vi "StartPlay.vi"(8 "error in (no error)":errorcluster, 11 "CameraTestingBL in":refnum<class "CameraTesting.lvclass">) -> (0 "error out":errorcluster, 3 "CameraTestingBL out":refnum<class "CameraTesting.lvclass">)   [LabVIEW 2020, in "CameraTesting.lvlib" / "CameraTesting.lvclass"]
doc: "Send command to camera to starting the data streaming"
uses:
  CameraTesting.lvclass
  CameraTesting.lvclass/CameraTesting.ctl
  <vilib>/ActorFramework/Message Enqueuer/Message Enqueuer.lvclass/Message Enqueuer.ctl
  <vilib>/ActorFramework/Message Enqueuer/Enqueue.vi
  ICameraTestingUI/ICameraTestingUI Messages/StartPlayRslt Msg/StartPlayRslt Msg.lvclass
  C:/Program Files (x86)/National Instruments/LabVIEW 2020/vi.lib/ActorFramework/Message/Message.lvclass
  <vilib>/ActorFramework/Message Priority Queue/Priority Enqueue.vi
  Camera/ICamera/ICamera/ICamera.lvclass
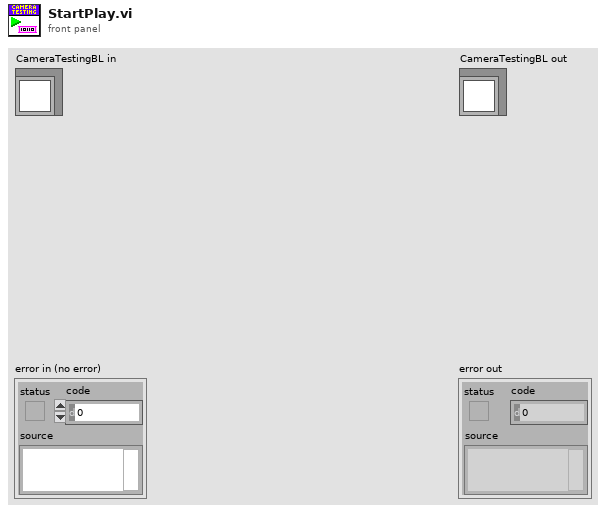
[diagram p1: front panel]
types:
  T1 = typedef "ICameraTesting.lvlib/ICameraTesting.lvclass/StatusUpdated.ctl" = refnum<user-event>
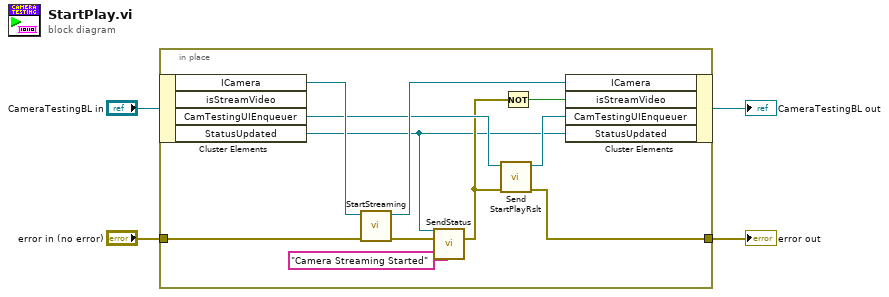
[diagram p0: block diagram]
diagram:
  n1 = in-place {
    in-place-border: "error in (no error)" -> [w15]
    in-place-border: [w10] -> w3
    n2 = in-place-cluster #1("CameraTestingBL in") -> ("ICamera"=w14:refnum<class "ICamera.lvclass">, "CamTestingUIEnqueuer"=w11:refnum<class "Message Enqueuer.lvclass">, "StatusUpdated"=w5:T1)  [unwired: 1 out]
    n3 = call-dynamic "StartStreaming.vi"("error in (no error)"=w15, "ICamera in"=w14) -> ("error out"=w7:errorcluster, "ICamera out"=w13:refnum<class "ICamera.lvclass">)  [unwired: 8 in]
    n4 = call "SendStatus.vi"("StatusUsrEvn"=w5, "error in"=w7, "Text"="Camera Streaming Started") -> ("error out"=w6:errorcluster)  [unwired: 24 in]
    n5 = call "Send StartPlayRslt.vi"("error in (no error)"=w6, "Message Enqueuer"=w11) -> ("error out"=w10:errorcluster, "Message Enqueuer out"=w9:refnum<class "Message Enqueuer.lvclass">)  [unwired: 8 in]
    n6 = Not(x=w6) -> (.not. x?=w12:bool)
    n7 = in-place-cluster #1("ICamera"=w13, "isStreamVideo"=w12, "CamTestingUIEnqueuer"=w9, "StatusUpdated"=w5) -> (→"CameraTestingBL out":refnum<class "CameraTesting.lvclass">)
  }
  "error out" <- w3
